vi "Read Measurement (Multiple).vi"(8 "error in (no error)":errorcluster, 10 "Timeout (10000 ms)":u32=10000, 11 "VISA resource name":refnum<visa-resource-name>) -> (0 "error out":errorcluster, 2 "Measurements":dbl[](array[numeric]) format="%#_12g", 3 "VISA resource name out":refnum<visa-resource-name>)   [LabVIEW 2024, in "Agilent 532XX Series.lvlib"]
doc: "Performs a single, new measurement and outputs multiple measurements."
uses:
  Agilent 532XX Series.lvlib
  Low Level/Fetch Measurement (Multiple).vi
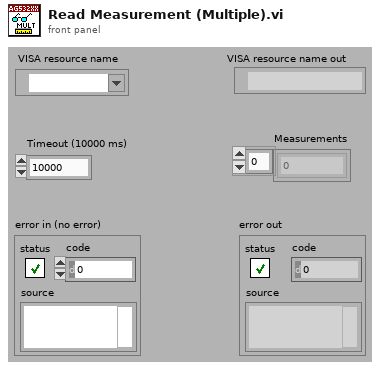
[diagram p1: front panel]
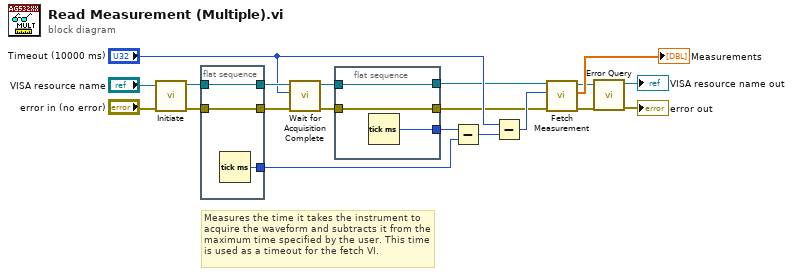
[diagram p0: block diagram]
diagram:
  # "Measures the time it takes the instrument to acquire the waveform and subtracts it from the maximum time specified by the user. This time is used as a timeout for the fetch VI."
  n1 = call "Initiate.vi"("error in (no error)"="error in (no error)", "VISA resource name"="VISA resource name") -> ("error out"=w14:errorcluster, "VISA resource name out"=w15:refnum<visa-resource-name>)  [unwired: 8 out]
  n2 = flat-sequence {
    tunnel: [w23] -> w11
    tunnel: w15 -> [w23]
    tunnel: [w22] -> w12
    tunnel: w14 -> [w22]
    tunnel: [w21] -> w13
    frame #0 {
      n3 = Tick Count (ms)() -> (millisecond timer value=w21:u32)
    }
  }
  n4 = call "Wait for Acquisition Complete.vi"("error in (no error)"=w12, "Maximum Time (10000 ms)"="Timeout (10000 ms)", "VISA resource name"=w11) -> ("error out"=w8:errorcluster, "VISA resource name out"=w9:refnum<visa-resource-name>)  [unwired: 1 in, 6 out]
  n5 = flat-sequence {
    tunnel: [w26] -> w4
    tunnel: w9 -> [w26]
    tunnel: [w25] -> w5
    tunnel: w8 -> [w25]
    tunnel: [w24] -> w7
    frame #0 {
      n6 = Tick Count (ms)() -> (millisecond timer value=w24:u32)
    }
  }
  n7 = Subtract(x=w7, y=w13) -> (x-y=w16:u32)
  n8 = Subtract(x="Timeout (10000 ms)", y=w16) -> (x-y=w6:u32)
  n9 = call-poly "Fetch Measurement.vi"("error in (no error)"=w5, "Timeout (10000 ms)"=w6, "VISA resource name"=w4) -> ("error out"=w1:errorcluster, "Measurements"=→"Measurements":dbl[], "VISA resource name out"=w2:refnum<visa-resource-name>)  [unwired: 6 out]
  n10 = call "Error Query.vi"("error in (no error)"=w1, "VISA resource name"=w2) -> ("error out"=→"error out":errorcluster, "VISA resource name out"=→"VISA resource name out":refnum<visa-resource-name>)  [unwired: 8 out]
